vi "DisplayScreen.vi"(8 "Grid":T2, 9 "square":T1, 11 "input picture":picture) -> (3 "2D Picture":picture)   [LabVIEW 2020]
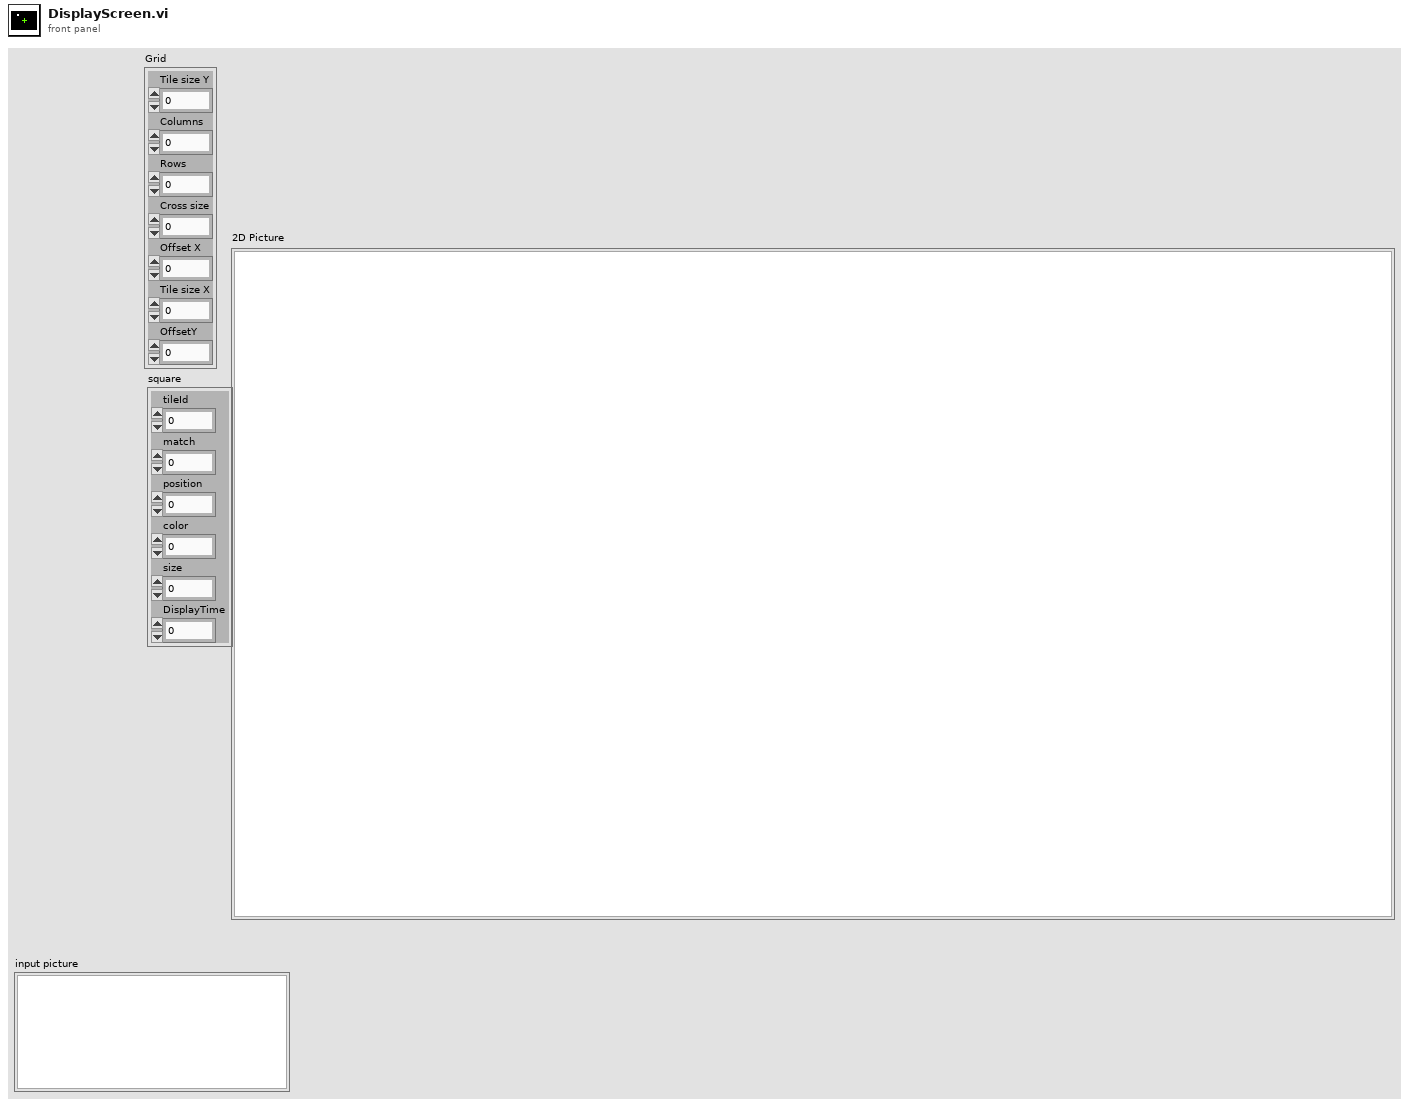
[diagram p1: front panel]
types:
  T1 = cluster{"tileId":i32, "match":i32, "position":i32, "color":u32, "size":i32, "DisplayTime":i32}
  T2 = cluster{"Tile size Y":dbl, "Columns":dbl, "Rows":dbl, "Cross size":dbl, "Offset X":dbl, "Tile size X":dbl, "OffsetY":dbl}
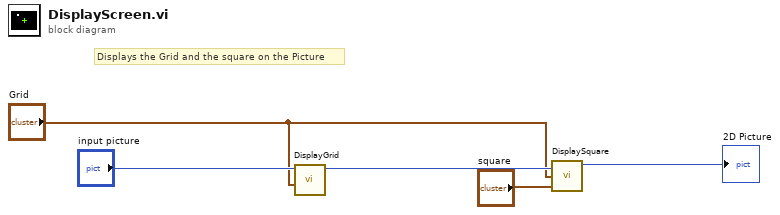
[diagram p0: block diagram]
diagram:
  # "Displays the Grid and the square on the Picture"
  n1 = call "DisplayGrid.vi"("Grid"="Grid", "input picture"="input picture") -> ("new picture"=w4:picture)  [unwired: 9 in]
  n2 = call "DisplaySquare.vi"("square"="square", "Grid"="Grid", "new picture in"=w4) -> ("new picture out"=→"2D Picture":picture)  [unwired: 5 in]
